vi "Set Echo Gate Colour [AG.EGT_COL].vi"(7 "Micropulse # In":i32, 8 "error in (no error)":errorcluster, 9 "Colour":u32(colorbox), 11 "Test Number":u32) -> (0 "error out":errorcluster, 5 "Micropulse # Out":i32)   [LabVIEW 2026, in "MicroPulse_Driver.lvlib"]
uses:
  MicroPulse_Driver.lvlib
  Private/MP-Registry Action-Enum.ctl
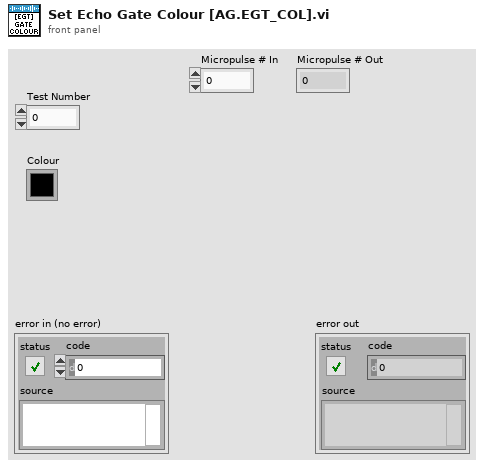
[diagram p1: front panel]
types:
  T1 = typedef "MicroPulse_Driver.lvlib/MP-Registry Action-Enum.ctl" = enum16{"Read", "Add Test", "Add Command", "Add Gate Command", "Add Encoder Command", "Clear Command  List", "Set Registry", "Set System Details", "Set DOF", "Set Velocity", "Disable Asynch Reads", "Enable Asynch Reads", "Add Connection", "Disconnect", "Shutdown"}
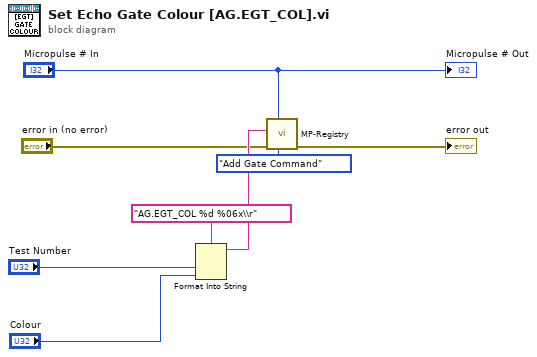
[diagram p0: block diagram]
diagram:
  n1 = Format Into String(format string="AG.EGT_COL %d %06x\\r", "Test Number", "Colour") -> (resulting string=w7:string)  [unwired: 2 in, 1 out]
  n2 = call "MP-Registry.vi"("Action"=MP-Registry_Action-Enum."Add Gate Command", "Micropulse # In"="Micropulse # In", "error in (no error)"="error in (no error)", "Data in"=w7) -> ("error out"=→"error out":errorcluster)  [unwired: 4 in, 3 out]
  "Micropulse # Out" <- "Micropulse # In"
